vi "1C Camera - Find Marker.vi"(8 "error in":errorcluster, 9 "Minimum Match Score (650)":sgl=650.0, 10 "marker template relative path":string="..\\1C Tracking Patterns\\4.5mm-BowMarker.png", 11 "Image In":T3(plugin-control)) -> (0 "error out":errorcluster, 1 "Best Match Position":cluster{"x":sgl, "y":sgl}, 2 "Best Match Heading":T1 format="%05.1f", 3 "Image Out":T3, 4 "Best Match\nBounding Box":cluster{"x":sgl, "y":sgl}[](array[cluster]), 5 "Marker found?":T2)   [LabVIEW 2011]
doc: "Finds a glyph in an image, and returns: a boolean of whether the glyph could be found, the location of the best match in the image, and its rotation from the glyph template.\n\nCoders: Cory, Gray and Jason\n\nRationale: For the Small RC platform, this is the VI that actually locates the two markers on the boat in an image, and returns their positions if they were found."
uses:
  <vilib>/vision/Image Controls.llb/IMAQ Image.ctl
  2-Think/2 Typedefs/indicator LED.ctl
  2-Think/2 Typedefs/heading.ctl
  <vilib>/vision/NI_Vision_Development_Module.lvlib
panel:
  in  "File Path":path
  out "Best Match":T4
  out "marker template absolute path":path
  out "Marker Template":T3(plugin-control)
  out "Matches":T5(array[cluster]) {"Bounding Box"."y" format="%.2f"; "Bounding Box"."x" format="%.2f"; "Position"."y" format="%.2f"; "Position"."x" format="%.2f"; "Score" format="%.2f"; "Scale" format="%.2f"; "Angle" format="%.2f"}
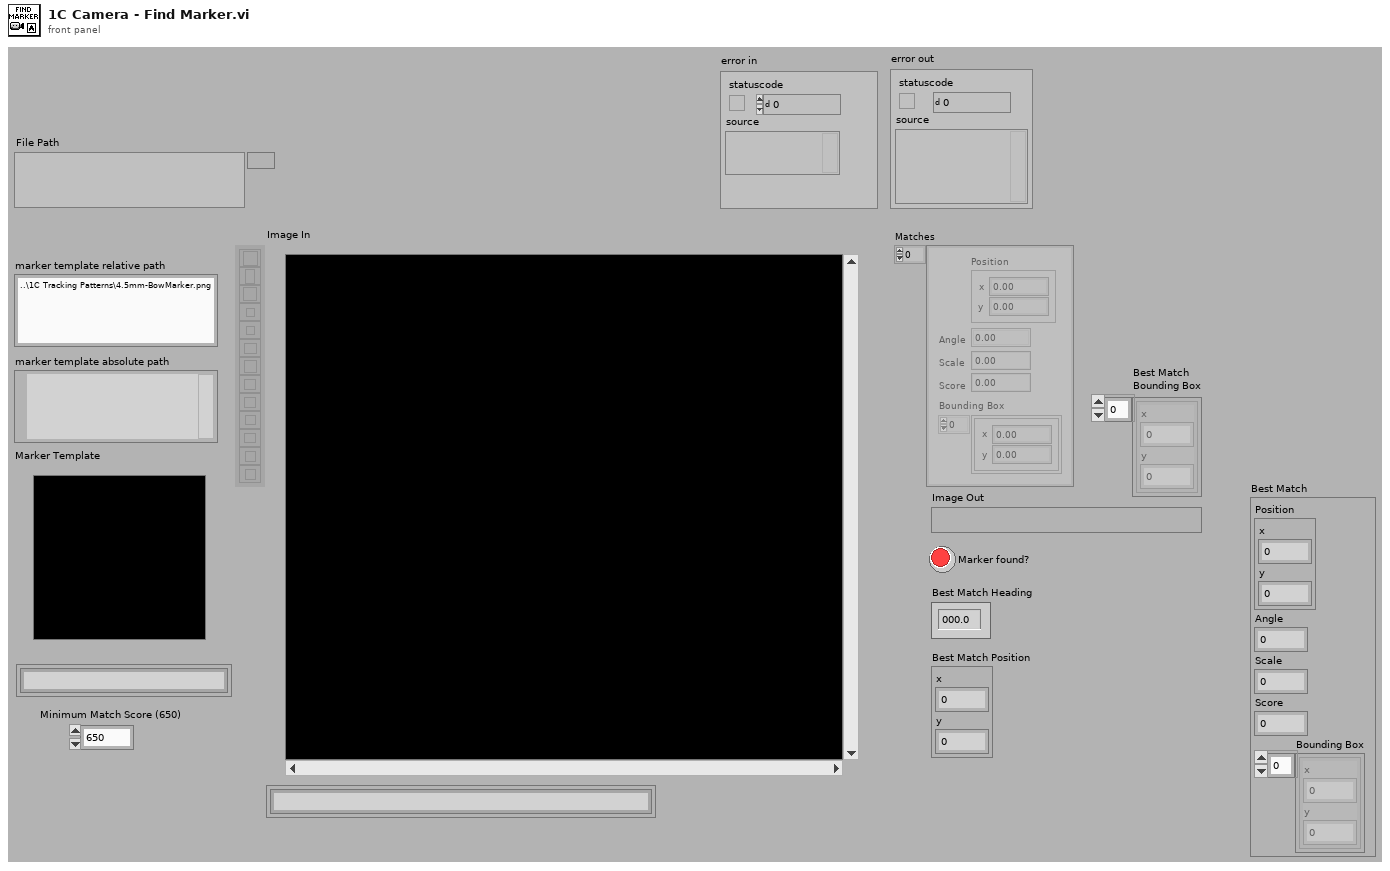
[diagram p1: front panel]
types:
  T1 = typedef "heading.ctl" = dbl
  T2 = typedef "indicator LED.ctl" = bool
  T3 = typedef "IMAQ Image.ctl" = refnum<image>
  T4 = cluster{"Position":cluster{"x":sgl, "y":sgl}, "Angle":sgl, "Scale":sgl, "Score":sgl, "Bounding Box":cluster{"x":sgl, "y":sgl}[]}
  T5 = cluster{"Position":cluster{"x":sgl, "y":sgl}, "Angle":sgl, "Scale":sgl, "Score":sgl, "Bounding Box":cluster{"x":sgl, "y":sgl}[]}[]
  T6 = typedef "Image Type" = u32
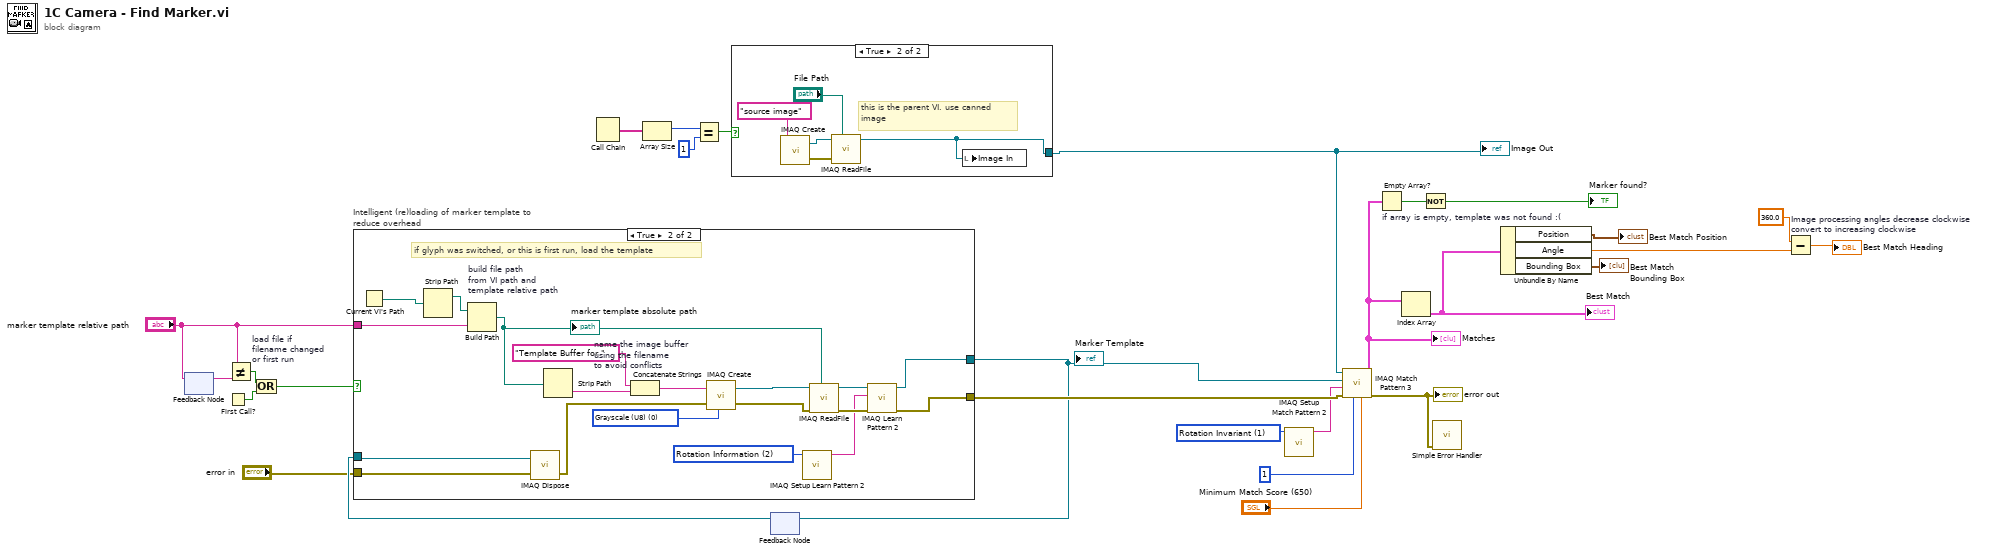
[diagram p0: block diagram]
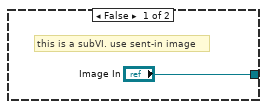
[diagram p2: hidden frame]
diagram:
  w12 = u16 1 items=["Shift Invariant", "Rotation Invariant"] ("Match Mode 2")
  n1 = feedback-in #1("marker template relative path") -> ()
  n2 = feedback #1() -> (w27:string)  [unwired: 1 in]
  n3 = First Call?() -> (First Call?: T/F=w24:bool)
  n4 = Not Equal?(x="marker template relative path", y=w27) -> (x != y?=w25:bool)
  n5 = Or "load file if\nfilename changed\nor first run"(x=w25, y=w24) -> (x .or. y?=w13:bool)
  n6 = Call Chain() -> (call chain=w4:string[])
  n7 = Array Size(array=w4) -> (size(s)=w6:i32)
  n8 = Equal?(x=w6, y=1) -> (x = y?=w3:bool)
  n9 = case shown="True" w3 {
    tunnel: ["Image In" w32] -> w2
    frame False {
      # "this is a subVI. use sent-in image"
    }
    frame True {
      # "this is the parent VI. use canned\nimage"
      n10 = call "IMAQ Create"("Image Name"="source image") -> ("New Image"=w34:T3, "error out"=w33:errorcluster)  [unwired: 4 in]
      n11 = call "IMAQ ReadFile"("File Path"="File Path", "error in (no error)"=w33, "Image"=w34) -> ("Image Out"=w32:T3)  [unwired: 4 in, 4 out]
      n12 = local write "Image In"(w32) -> ()
    }
  }
  "Image Out" <- w2
  n13 = feedback #2() -> (w26:T3)  [unwired: 1 in]
  n14 = case "Intelligent (re)loading of marker template to reduce overhead" shown="True" w13 {
    tunnel: [w36 w41] -> w14
    tunnel: "marker template relative path" -> [_ w51]
    tunnel: w26 -> [w36 w50]
    tunnel: [w35 w39] -> w19
    tunnel: "error in" -> [w35 w48]
    frame False {
      # "if the path has not changed,\njust keep the same template from last time"
    }
    frame True {
      w38 = u16 2 items=["All", "Shift Information", "Rotation Information"] ("Learn Mode")
      w54 = T6 0 items=["Grayscale (U8)", "Grayscale (I16)", "Grayscale (SGL)", "Complex (CSG)", "RGB (U32)", "HSL (U32)", "RGB (U64)", "Grayscale (U16)"] ("Image Type")
      # "if glyph was switched, or this is first run, load the template"
      n15 = Current VI's Path() -> (path=w53:path)
      n16 = Strip Path(path=w53) -> (stripped path=w52:path)  [unwired: 1 out]
      n17 = Build Path "build file path\nfrom VI path and \ntemplate relative path"(base path=w52, name or relative path=w51) -> (appended path=w45:path)
      "marker template absolute path" <- w45
      n18 = call "IMAQ Dispose"("Image"=w50, "error in (no error)"=w48) -> ("error out"=w47:errorcluster)  [unwired: 4 in]
      n19 = Strip Path(path=w45) -> (name=w43:string)  [unwired: 1 out]
      n20 = Concatenate Strings "name the image buffer\nusing the filename\nto avoid conflicts"("Template Buffer for " ("Image Name"), w43) -> (w46:string)
      n21 = call "IMAQ Create"("Image Name"=w46, "Image Type"=w54, "error in (no error)"=w47) -> ("New Image"=w55:T3, "error out"=w49:errorcluster)  [unwired: 2 in]
      n22 = call "IMAQ Setup Learn Pattern 2"("Learn Mode"=w38) -> ("Learn Pattern Setup Data"=w37:string)  [unwired: 9 in, 1 out]
      n23 = call "IMAQ ReadFile"("File Path"=w45, "error in (no error)"=w49, "Image"=w55) -> ("error out"=w40:errorcluster, "Image Out"=w42:T3)  [unwired: 4 in, 3 out]
      n24 = call "IMAQ Learn Pattern 2"("error in (no error)"=w40, "Learn Pattern Setup Data"=w37, "Image"=w42) -> ("error out"=w39:errorcluster, "Template Image Out"=w41:T3)  [unwired: 7 in]
    }
  }
  "Marker Template" <- w14
  n25 = feedback-in #2(w14) -> ()
  n26 = call "IMAQ Setup Match Pattern 2"("Match Mode"=w12) -> ("Match Pattern Setup Data"=w9:string)  [unwired: 9 in, 1 out]
  n27 = call "IMAQ Match Pattern 3"("Minimum Match Score"="Minimum Match Score (650)", "Number of Matches Requested"=1, "error in (no error)"=w19, "Match Pattern Setup Data"=w9, "Template Image"=w14, "Image"=w2) -> ("error out"=w7:errorcluster, "Matches"=w8:T5)  [unwired: 3 in, 1 out]
  "Matches" <- w8
  "error out" <- w7
  n28 = Empty Array? "if array is empty, template was not found :("(array=w8) -> (empty?=w21:bool)
  n29 = Index Array(array=w8) -> (element=w23:T4)  [unwired: 1 in]
  "Best Match" <- w23
  n30 = Not(x=w21) -> (.not. x?=→"Marker found?":bool)
  n31 = call <vilib>:"Simple Error Handler.vi"("error in (no error)"=w7) -> ()  [unwired: 4 in, 5 out]
  n32 = Unbundle By Name(w23) -> ("Position"=→"Best Match Position":cluster{"x":sgl, "y":sgl}, "Angle"=w16:sgl, "Bounding Box"=→"Best Match\nBounding Box":cluster{"x":sgl, "y":sgl}[])
  n33 = Subtract "Image processing angles decrease clockwise\nconvert to increasing clockwise"(x=sgl 360.0 ("y"), y=w16) -> (x-y=→"Best Match Heading":sgl)
